vi "Is Transmit Ready.vi"(8 "error in (no error)":errorcluster, 10 "Samples to transmit":i32=1024, 11 "RP Lockin in":refnum<class "RP Transceiver.lvclass">) -> (0 "error out":errorcluster, 2 "Transmit Ready":bool, 3 "RP Lockin out":refnum<class "RP Transceiver.lvclass">)   [LabVIEW 2015, in "RP Transceiver.lvclass"]
uses:
  RP Transceiver.lvclass
  RP Transceiver.lvclass/RP Transceiver.ctl
  RP Communicator/RP Communicator.lvclass
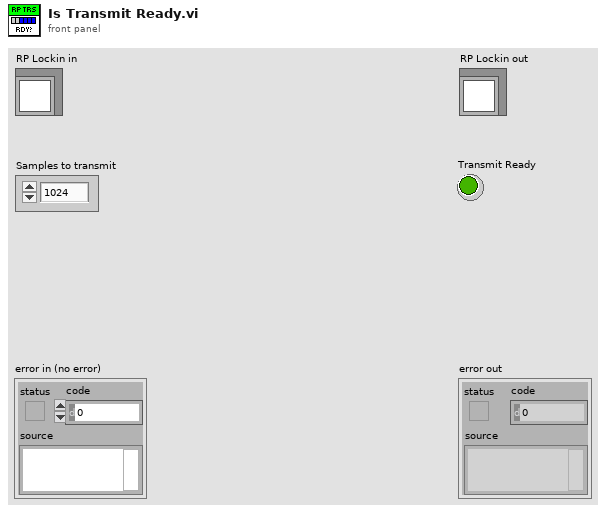
[diagram p1: front panel]
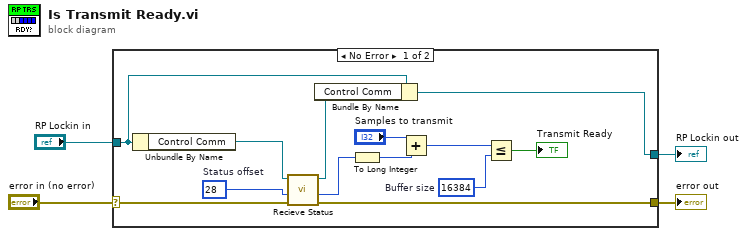
[diagram p0: block diagram]
diagram:
  n1 = case shown="No Error" "error in (no error)" {
    selector: "error in (no error)" -> [w10 w19]
    tunnel: [w9 w19] -> w3
    tunnel: [w12 w18] -> w1
    tunnel: "RP Lockin in" -> [w17 w18]
    frame No Error {
      w6 = 16384  # Buffer size
      w15 = u64 28  # Status offset
      n2 = Unbundle By Name(w17) -> ("Control Comm"=w16:refnum<class "RP Communicator.lvclass">)
      n3 = call-dynamic "Recieve Status.vi"("error in (no error)"=w10, "Status offset"=w15, "RP Communicator in"=w16) -> ("error out"=w9:errorcluster, "Status response"=w14:u32, "RP Communicator out"=w11:refnum<class "RP Communicator.lvclass">)  [unwired: 6 in]
      n4 = Bundle By Name(cluster=w17, "Control Comm"=w11) -> (w12:refnum<class "RP Transceiver.lvclass">)
      n5 = To Long Integer(number=w14) -> (32bit integer=w8:i32)
      n6 = Add(x="Samples to transmit", y=w8) -> (x+y=w5:i32)
      n7 = Less Or Equal?(x=w5, y=w6) -> (x <= y?=→"Transmit Ready":bool)
    }
    frame Error {
    }
  }
  "error out" <- w3
  "RP Lockin out" <- w1
